vi "Match Beacon.vi"(8 "Known Beacon":cluster{"X":i64, "Y":i64, "Z":i64}, 9 "Known Beacons":cluster{"X":i64, "Y":i64, "Z":i64}[](array[cluster]), 10 "Unknown Beacon":cluster{"X":i64, "Y":i64, "Z":i64}, 11 "Unknown Beacons":cluster{"X":i64, "Y":i64, "Z":i64}[](array[cluster])) -> (1 "Scanner Position":cluster{"X":i64, "Y":i64, "Z":i64}, 2 "Match?":bool, 3 "New Beacons":cluster{"X":i64, "Y":i64, "Z":i64}[](array[cluster]))   [LabVIEW 2021]
uses:
  d0df36b0-5b2c-41f6-b463-2c426b41e130.vi
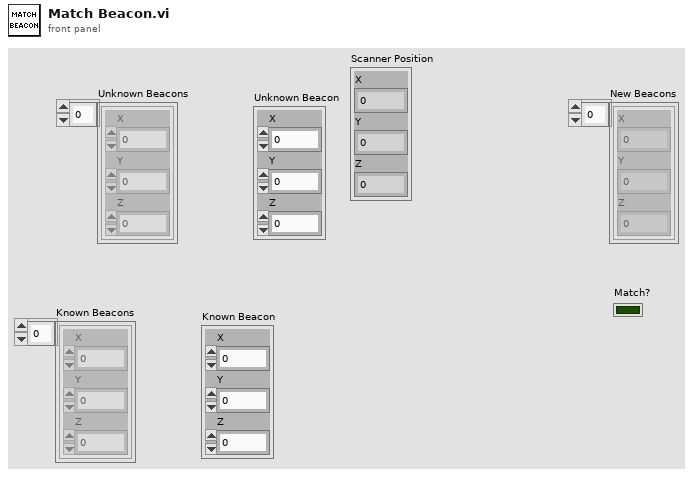
[diagram p1: front panel]
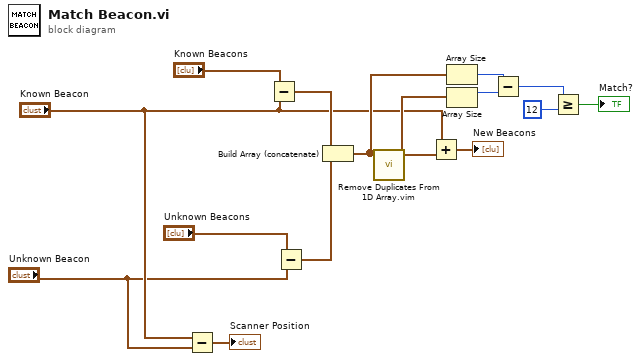
[diagram p0: block diagram]
diagram:
  n1 = Subtract(x="Known Beacon", y="Unknown Beacon") -> (x-y=→"Scanner Position":cluster{"X":i64, "Y":i64, "Z":i64})
  n2 = Subtract(x="Known Beacons", y="Known Beacon") -> (x-y=w10:cluster{"X":i64, "Y":i64, "Z":i64}[])
  n3 = Subtract(x="Unknown Beacons", y="Unknown Beacon") -> (x-y=w11:cluster{"X":i64, "Y":i64, "Z":i64}[])
  n4 = Build Array (concatenate)(w10, w11) -> (w9:cluster{"X":i64, "Y":i64, "Z":i64}[])
  n5 = call "Remove Duplicates From 1D Array.vim"("array"=w9) -> ("array with duplicates removed"=w5:cluster{"X":i64, "Y":i64, "Z":i64}[])  [unwired: 10 in]
  n6 = Add(x="Known Beacon", y=w5) -> (x+y=→"New Beacons":cluster{"X":i64, "Y":i64, "Z":i64}[])
  n7 = Array Size(array=w9) -> (size(s)=w8:i32)
  n8 = Array Size(array=w5) -> (size(s)=w7:i32)
  n9 = Subtract(x=w8, y=w7) -> (x-y=w6:i32)
  n10 = Greater Or Equal?(x=w6, y=12) -> (x >= y?=→"Match?":bool)
